vi "Write Find Fiducials.vi"(8 "error in":errorcluster, 10 "Find Fiducials":T1, 11 "Potting Procedure in":refnum<class "Potting Procedure.lvclass">) -> (0 "error out":errorcluster, 3 "Potting Procedure out":refnum<class "Potting Procedure.lvclass">)   [LabVIEW 2011, in "Potting Procedure.lvclass"]
uses:
  Potting Procedure.lvclass
  Type Definitions/Inspect Fiducials.ctl
  Shared Components/Utils/Type Definitions/Fiducial Image.ctl
  Shared Components/Vec3d Class/Vec3d Class.lvclass
  Shared Components/Utils/Type Definitions/Physical Image.ctl
  <vilib>/vision/Image Controls.llb/IMAQ Image.ctl
  Shared Components/Utils/Type Definitions/Fiducial with Source.ctl
  Potting Procedure.lvclass/Potting Procedure.ctl
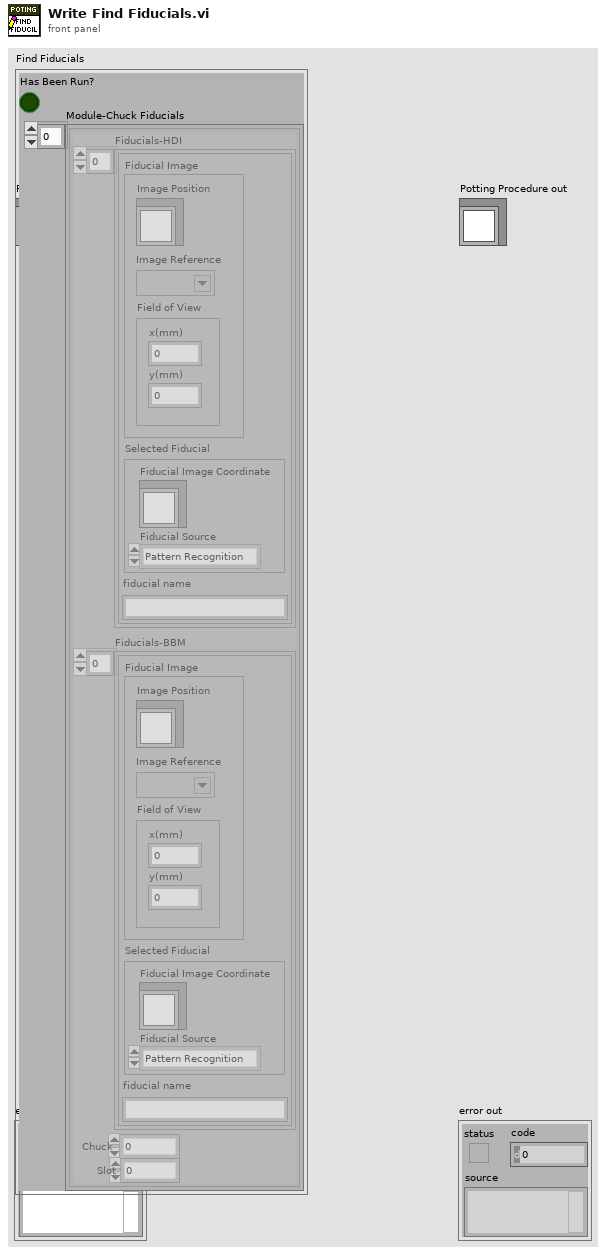
[diagram p1: front panel]
types:
  T1 = typedef "Inspect Fiducials.ctl" = cluster{"Has Been Run?":bool, "Module-Chuck Fiducials":cluster{"Fiducials-HDI":T2[], "Fiducials-BBM":T2[], "Chuck":i32, "Slot":i32}[]}
  T2 = typedef "Fiducial Image.ctl" = cluster{"Fiducial Image":T3, "Selected Fiducial":T5, "fiducial name":string}
  T3 = typedef "Physical Image.ctl" = cluster{"Image Position":refnum<class "Vec3d Class.lvclass">, "Image Reference":T4, "Field of View":cluster{"x(mm)":dbl, "y(mm)":dbl}}
  T4 = typedef "IMAQ Image.ctl" = refnum<image>
  T5 = typedef "Fiducial with Source.ctl" = cluster{"Fiducial Image Coordinate":refnum<class "Vec3d Class.lvclass">, "Fiducial Source":enum16{"Pattern Recognition", "User", "Error", "Default"}}
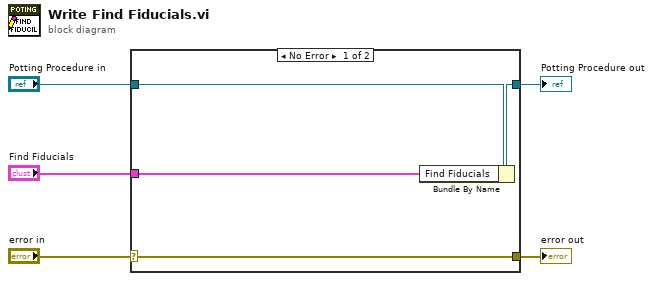
[diagram p0: block diagram]
diagram:
  n1 = case shown="No Error" "error in" {
    selector: "error in" -> [w9 w10]
    tunnel: [w9 w10] -> w4
    tunnel: [w7 w11] -> w2
    tunnel: "Potting Procedure in" -> [w8 w11]
    tunnel: "Find Fiducials" -> [w6 _]
    frame No Error {
      n2 = Bundle By Name(cluster=w8, "Find Fiducials"=w6) -> (w7:refnum<class "Potting Procedure.lvclass">)
    }
    frame Error {
    }
  }
  "error out" <- w4
  "Potting Procedure out" <- w2
